vi "calc_scanner_pos.vi"(8 "error in (no error)":errorcluster, 10 "Draw Area Size":T1, 11 "Mouse position":cluster{"X":i32, "Y":i32}) -> (0 "error out":errorcluster, 3 "Scanner position":dbl[](array[numeric]))   [LabVIEW 2010]
uses:
  <vilib>/Utility/miscctls.llb/LVBoundsTypeDef.ctl
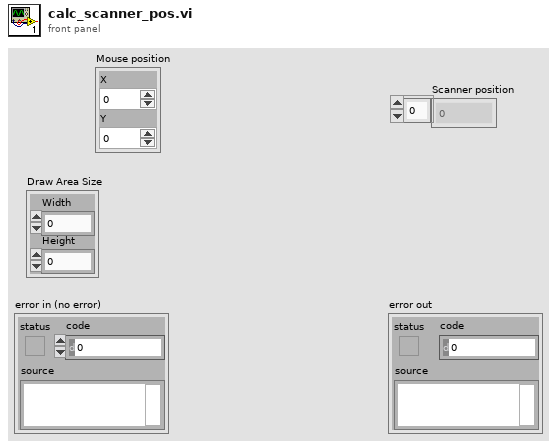
[diagram p1: front panel]
types:
  T1 = typedef "LVBoundsTypeDef.ctl" = cluster{"Width":u32, "Height":u32}
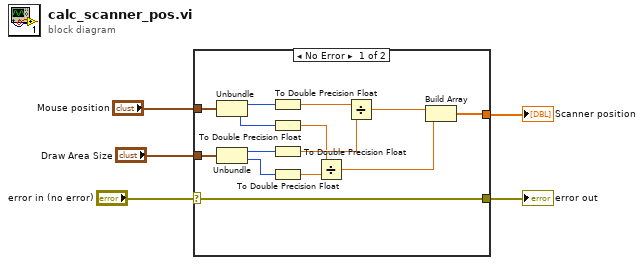
[diagram p0: block diagram]
diagram:
  n1 = case shown="No Error" "error in (no error)" {
    selector: "error in (no error)" -> [w19 w20]
    tunnel: [w19 w20] -> w4
    tunnel: "Draw Area Size" -> [w18 _]
    tunnel: "Mouse position" -> [w17 _]
    tunnel: [w6 _] -> w1
    frame No Error {
      n2 = Unbundle(w17) -> ("X"=w14:i32, "Y"=w13:i32)
      n3 = Unbundle(w18) -> ("Width"=w16:u32, "Height"=w15:u32)
      n4 = To Double Precision Float(number=w14) -> (double precision float=w12:dbl)
      n5 = To Double Precision Float(number=w13) -> (double precision float=w10:dbl)
      n6 = To Double Precision Float(number=w16) -> (double precision float=w11:dbl)
      n7 = To Double Precision Float(number=w15) -> (double precision float=w9:dbl)
      n8 = Divide(x=w10, y=w9) -> (x/y=w7:dbl)
      n9 = Divide(x=w12, y=w11) -> (x/y=w8:dbl)
      n10 = Build Array(w8, w7) -> (w6:dbl[])
    }
    frame Error {
    }
  }
  "error out" <- w4
  "Scanner position" <- w1
